vi "PlotDrag-Mouse Move.vi"(0 "Drag State In":T1, 5 "XYGraph in":refnum<vi>, 7 "Coords":T2, 11 "error in (no error)":errorcluster) -> (4 "Drag State Out":T1, 15 "error out":errorcluster)   [LabVIEW 2020]
uses:
  PlotDrag-State.ctl
  <vilib>/Utility/miscctls.llb/LVPoint32TypeDef.ctl
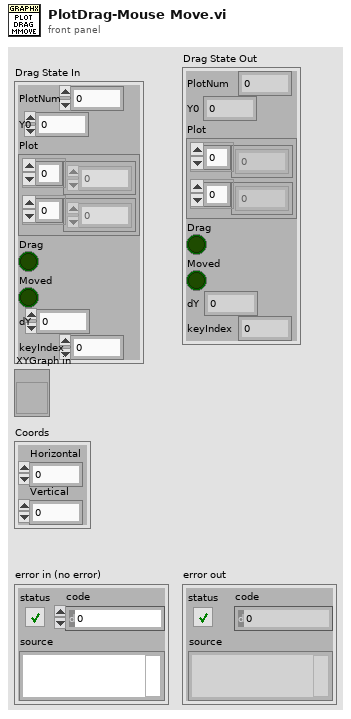
[diagram p1: front panel]
types:
  T1 = typedef "PlotDrag-State.ctl" = cluster{"PlotNum":i32, "Y0":dbl, "Plot":cluster{dbl[], dbl[]}, "Drag":bool, "Moved":bool, "dY":dbl, "keyIndex":i32}
  T2 = typedef "LVPoint32TypeDef.ctl" = cluster{"Horizontal":i32, "Vertical":i32}
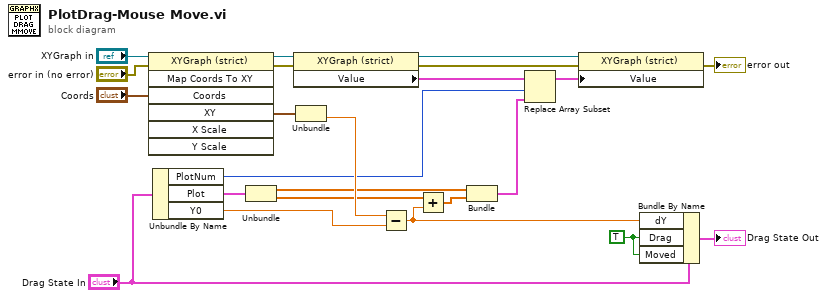
[diagram p0: block diagram]
diagram:
  w2 = TRUE ("Dragging")
  n1 = invoke class="XYGraph (strict)" method="Map Coords To XY"(reference="XYGraph in", error in="error in (no error)", "Coords"="Coords") -> (reference out=w12:refnum<vi>, error out=w11:errorcluster, "XY"=w21:cluster{"X":dbl, "Y":dbl})  [unwired: 4 in, 4 out]
  n2 = Unbundle By Name("Drag State In") -> ("PlotNum"=w10:i32, "Plot"=w16:cluster{dbl[], dbl[]}, "Y0"=w13:dbl)
  n3 = Unbundle(w16) -> (w15:dbl[], w14:dbl[])
  n4 = property class="XYGraph (strict)"(reference=w12, error in=w11) -> (reference out=w6:refnum<vi>, error out=w7:errorcluster, "Value"=w9:cluster{dbl[], dbl[]}[])
  n5 = Unbundle(w21) -> ("Y"=w20:dbl)  [unwired: 1 out]
  n6 = Subtract(x=w20, y=w13) -> (x-y=w1:dbl)
  n7 = Add(x=w14, y=w1) -> (x+y=w19:dbl[])
  n8 = Bundle(w15, w19) -> (w18:cluster{dbl[], dbl[]})  [unwired: 1 in]
  n9 = Replace Array Subset(array=w9, new element=w18, index=w10) -> (w8:cluster{dbl[], dbl[]}[])
  n10 = property class="XYGraph (strict)"(reference=w6, error in=w7, "Value"=w8) -> (error out=→"error out":errorcluster)  [unwired: 1 out]
  n11 = Bundle By Name(cluster="Drag State In", "dY"=w1, "Drag"=w2, "Moved"=w2) -> (→"Drag State Out":T1)
